vi "ST_1_PRCC_BY_LabV_TO_PLC.vi"(7 "Enum":enum16{"Read", "Write"}(ring), 8 "error in (no error)":errorcluster, 11 "ST 1 DATA":i64[](array[numeric])) -> (0 "error out":errorcluster, 3 "ST 1 DATA OUT":i64[](array[numeric]))   [LabVIEW 2017]
panel:
  # "CONTROL PROCESS TO PLC FROM LABVIEW"
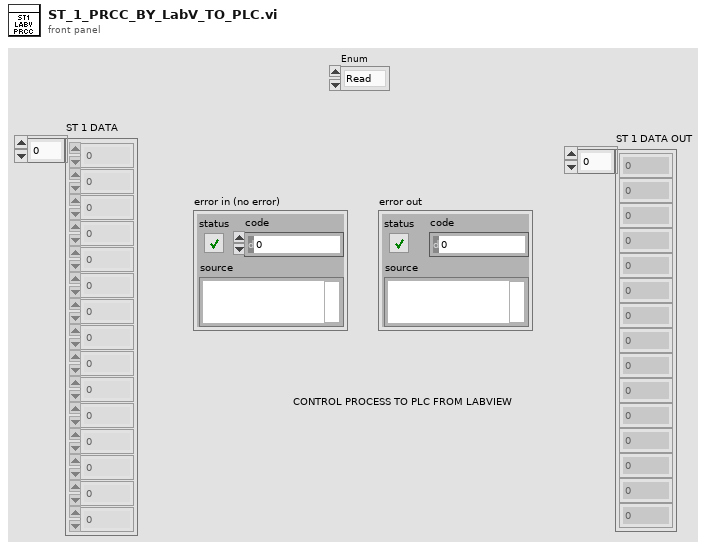
[diagram p1: front panel]
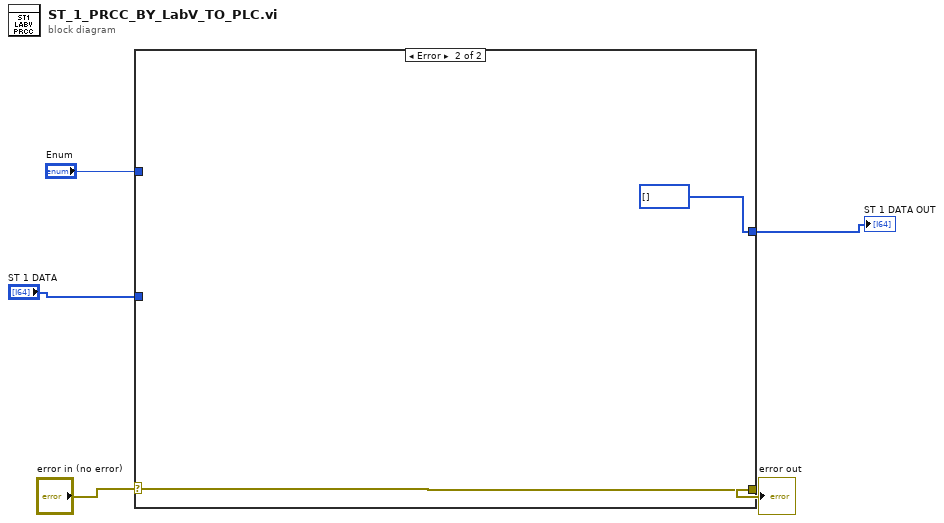
[diagram p0: block diagram]
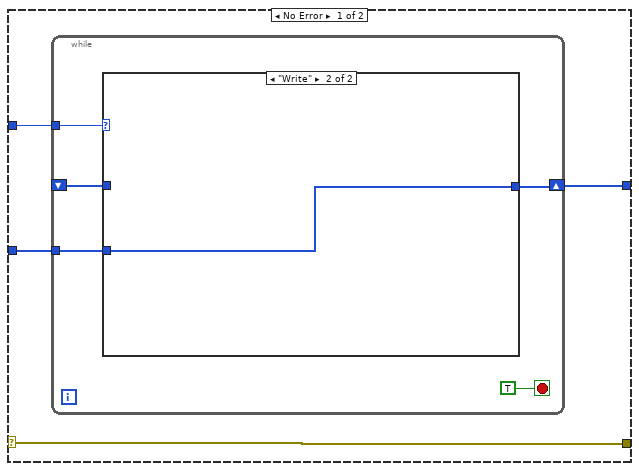
[diagram p2: hidden frame]
diagram:
  n1 = case shown="Error" "error in (no error)" {
    selector: "error in (no error)" -> [w6 w18]
    tunnel: [w6 w18] -> w5
    tunnel: "Enum" -> [w9 _]
    tunnel: "ST 1 DATA" -> [w8 _]
    tunnel: [w7 i64[] [] ("ST 1 DATA")] -> w1
    frame No Error {
      n2 = while {
        tunnel: w9 -> [w13]
        shift-right: [w10] -> w7
        shift-left: _ -> [w11]
        tunnel: w8 -> [w12]
        stop <- TRUE stop-if-true
        n3 = case shown="\"Write\"" w13 {
          tunnel: w12 -> [_ w16]
          tunnel: [w15 w16] -> w10
          tunnel: w11 -> [w15 _]
          frame "Read", Default {
          }
          frame "Write" {
          }
        }
      }
    }
    frame Error {
    }
  }
  "error out" <- w5
  "ST 1 DATA OUT" <- w1
